vi "generateXML.vi"(7 "attributeString":string, 8 "error in":errorcluster, 9 "childrenXML":string[](array[string]), 10 "elementName":string, 11 "WriteElement in":refnum<class "XMLGenerator.lvclass">) -> (0 "error out":errorcluster, 2 "XML out":string, 3 "WriteElement out":refnum<class "XMLGenerator.lvclass">)   [LabVIEW 2016, in "XML.lvlib" / "XMLGenerator.lvclass"]
doc: "The main, public, method for XML generation that takes the element name and any chlidren contents and creates a fully formatted XML string."
uses:
  <userlib>/Common/XML/XMLGenerator/XMLGenerator.lvclass
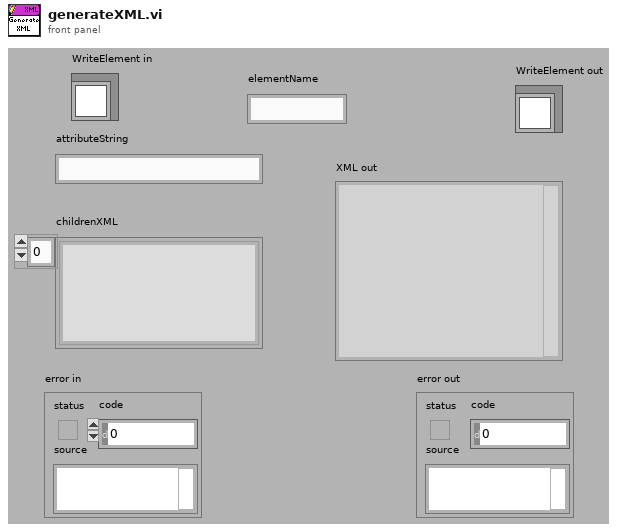
[diagram p1: front panel]
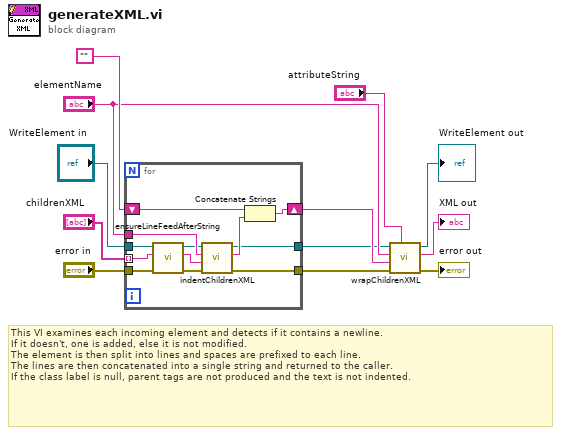
[diagram p0: block diagram]
diagram:
  # "This VI examines each incoming element and detects if it contains a newline.\nIf it doesn't, one is added, else it is not modified.  \nThe element is then split into lines and spaces are prefixed to each line.  \nThe lines are then concatenated into a single string and returned to the caller. \nIf the class label is null, parent tags are not produced and the text is not indented."
  n1 = for {
    tunnel: "childrenXML" -> [w23] mode=indexing
    tunnel: "error in" -> [w22]
    tunnel: [w17] -> w6
    shift-right: [w24] -> w8
    shift-left: "" -> [w20]
    tunnel: "elementName" -> [w21]
    tunnel: "WriteElement in" -> [w16]
    tunnel: [w14] -> w2
    n2 = call <userlib>:"ensureLineFeedAfterString.vi"("error in (no error)"=w22, "Element"=w23, "WriteElement in"=w16) -> ("error out"=w18:errorcluster, "ElementWithNewLine"=w13:string, "WriteElement out"=w15:refnum<class "XMLGenerator.lvclass">)  [unwired: 6 in]
    n3 = call <userlib>:"indentChildrenXML.vi"("error in (no error)"=w18, "childXML"=w13, "parentElementName"=w21, "WriteElement in"=w15) -> ("error out"=w17:errorcluster, "indentedChildrenXML"=w19:string, "WriteElement out"=w14:refnum<class "XMLGenerator.lvclass">)  [unwired: 5 in]
    n4 = Concatenate Strings(w20, w19) -> (w24:string)
  }
  n5 = call <userlib>:"wrapChildrenXML.vi"("parentAttributeString"="attributeString", "error in (no error)"=w6, "childrenXML"=w8, "parentName"="elementName", "WriteElement in"=w2) -> ("error out"=→"error out":errorcluster, "XML out"=→"XML out":string, "WriteElement out"=→"WriteElement out":refnum<class "XMLGenerator.lvclass">)  [unwired: 4 in]
